vi "Get LoopTunnel Terminals Datatypes.vi"(8 "Error In":errorcluster, 10 "Outer Terminal":refnum<vi>, 11 "Inner Terminals[]":refnum<vi>[](array[refnum])) -> (0 "Error Out":errorcluster, 2 "Outer Terminal Datatype":string[](array[string]), 3 "Inner Terminals Datatypes [][]":string[][](array[string]))   [LabVIEW 2018]
doc: "Returns datatypes of inner terminals and outer terminal."
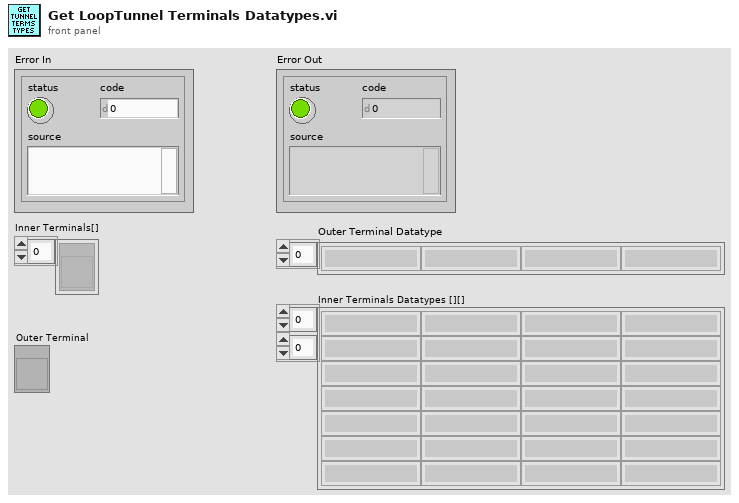
[diagram p1: front panel]
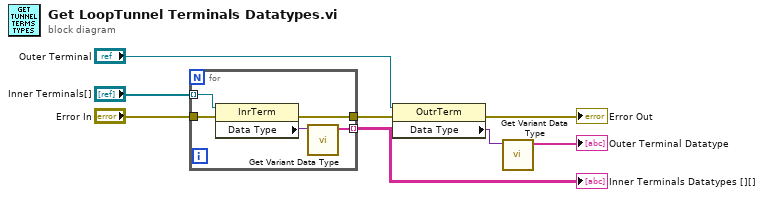
[diagram p0: block diagram]
diagram:
  n1 = for {
    tunnel: [w12] -> w1 mode=indexing
    tunnel: "Inner Terminals[]" -> [w11] mode=indexing
    tunnel: "Error In" -> [w10]
    tunnel: [w9] -> w6
    n2 = property class="InrTerm"(reference=w11, error in=w10) -> (error out=w9:errorcluster, "Data Type"=w13:variant)  [unwired: 1 out]
    n3 = call "Get Variant Data Type.vi"("Variant in"=w13) -> ("Data Types[]"=w12:string[])  [unwired: 9 in, 1 out]
  }
  "Inner Terminals Datatypes [][]" <- w1
  n4 = property class="OutrTerm"(reference="Outer Terminal", error in=w6) -> (error out=→"Error Out":errorcluster, "Data Type"=w4:variant)  [unwired: 1 out]
  n5 = call "Get Variant Data Type.vi"("Variant in"=w4) -> ("Data Types[]"=→"Outer Terminal Datatype":string[])  [unwired: 9 in, 1 out]
